vi "Close Adu232.vi"(8 "error in (no error)":errorcluster, 11 "RS232 handle":u32) -> (0 "error out":errorcluster)   [LabVIEW 2015, in "AduHid.lvlib"]
doc: "void __stdcall CloseAdu232(void * hRS232);"
uses:
  AduHid.lvlib
  AduHid.dll
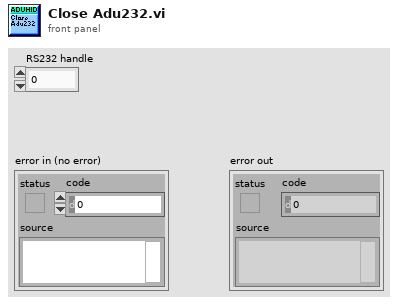
[diagram p1: front panel]
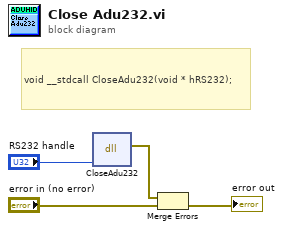
[diagram p0: block diagram]
diagram:
  # "void __stdcall CloseAdu232(void * hRS232);"
  n1 = dll-call lib="C:/Projects/CBTF Modules/Libraries/Ontrak ADU/API/AduHid.*" fn="CloseAdu232"("RS232 handle"="RS232 handle") -> (error out=w2:errorcluster)  [unwired: 5 in, 1 out]
  n2 = Merge Errors(w2, "error in (no error)") -> (→"error out":errorcluster)
